vi "求阶乘.vi"(11 "Num":i32=100) -> (3 "Fract":dbl)   [LabVIEW 2011]
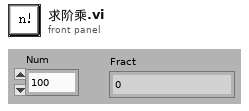
[diagram p1: front panel]
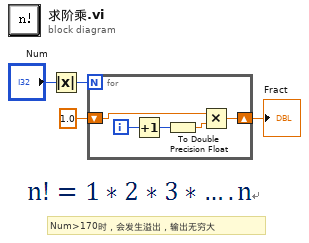
[diagram p0: block diagram]
diagram:
  # "Num>170时，会发生溢出，输出无穷大"
  n1 = Absolute Value(x="Num") -> (abs(x)=w3:i32)
  n2 = for {
    N: w3 -> [_]
    shift-right: [w6] -> w1
    shift-left: 1.0 -> [w7]
    i -> [w9]
    n3 = Increment(x=w9) -> (x+1=w8:i32)
    n4 = To Double Precision Float(number=w8) -> (double precision float=w5:dbl)
    n5 = Multiply(x=w7, y=w5) -> (x*y=w6:dbl)
  }
  "Fract" <- w1
